vi "Create Frame Pattern Script.vi"(8 "error in (no error)":errorcluster, 10 "SPI_FRM_Config":T1 {"Addr" format="%x"; "Data" format="%x"}, 11 "SPI_Frame_Write in":refnum<class "SPI_Frame_Write.lvclass">) -> (0 "error out":errorcluster, 3 "SPI_Frame_Write out":refnum<class "SPI_Frame_Write.lvclass">)   [LabVIEW 2018, in "SPI_Frame_Write.lvclass"]
uses:
  SPI_Frame_Write.lvclass
  C:/P4 Workspace/PC Client/Solutions/5g_eap/HiSi/trunk/1.0/BML_Pattern_Gen_Refactor/SPI/SPI Frame Root/SPI_Frame_Root.lvclass
  Config Read SPI/SPI_FRM_Config.ctl
  Classes/Config_Read/RW_Option.ctl
  Config Read SPI/SPI_Mode.ctl
  SPI Frame Root/DataType.ctl
  Classes/BML_Frame_Root/Special Frame.ctl
  SPI Frame Root/SPI_Frame_Root.lvclass/SPI_Frame_Root.ctl
  Classes/BML_Frame_Root/BML_Frame_Root.lvclass
  SPI Frame Root/SPI_Frame_Root.lvclass
  Classes/Config_Read/Config_Read_BML.lvclass
  Config Read SPI/Config_Read_SPI.lvclass
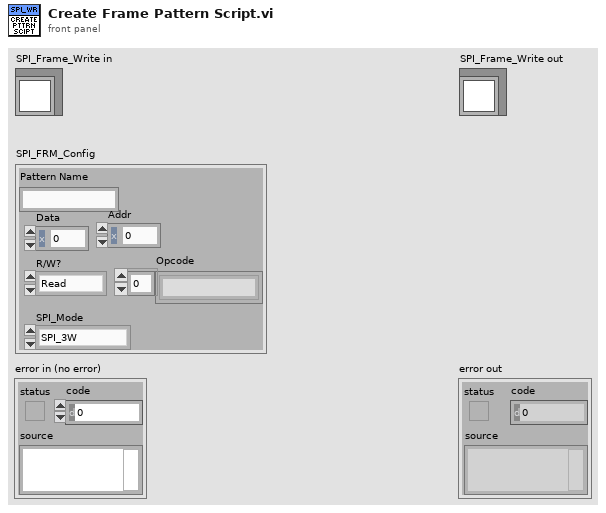
[diagram p1: front panel]
types:
  T1 = typedef "Config_Read_SPI.lvclass/SPI_FRM_Config.ctl" = cluster{"Pattern Name":string, "Data":u16, "Addr":u16, "R/W?":T2, "Opcode":string[], "SPI_Mode":T3}
  T2 = typedef "Config_Read_BML.lvclass/RW_Option.ctl" = enum16{"Read", "Write", "R/W"}
  T3 = typedef "Config_Read_SPI.lvclass/SPI_Mode.ctl" = enum16{"SPI_3W", "SPI_4W"}
  T4 = typedef "BML_Frame_Root.lvclass/Special Frame.ctl" = enum16{"Sync Header", "Protocol Header", "SW Trig", "SetID State", "Out SetID State", "SW Reset", "Wait", "SPI 4W FRM Start", "SPI 4W Wait", "SPI 4W FRM End", "SPI 4W Write Cmd", "SPI RD Collect Cmd", "SPI RD Value Cmd", "SPI 3W FRM Start", "SPI 3W Write Cmd", "SPI 3W FRM End", "SPI 3W Wait", "SPI 3W RD Cmd"}
  T5 = typedef "SPI_Frame_Root.lvclass/DataType.ctl" = enum16{"Drive", "Compare", "Read"}
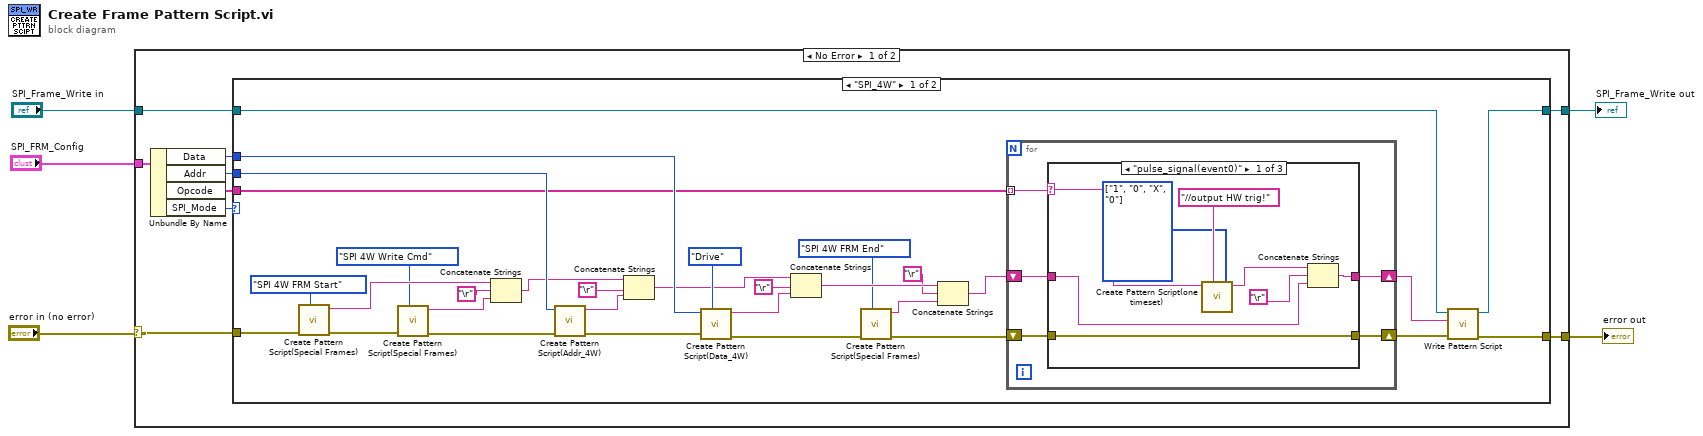
[diagram p0: block diagram]
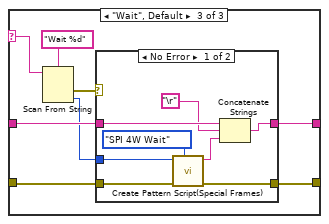
[diagram p3: hidden frame]
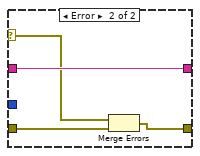
[diagram p4: hidden frame]
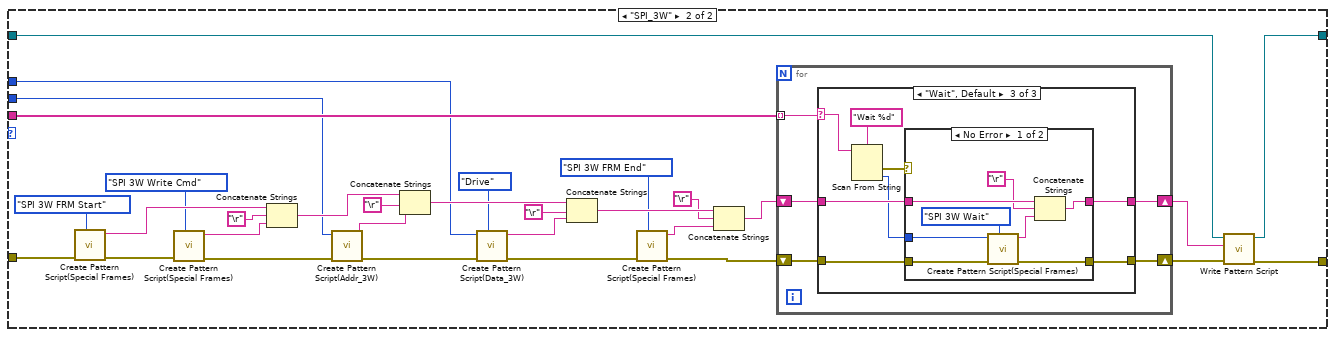
[diagram p5: hidden frame]
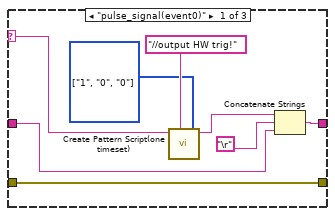
[diagram p6: hidden frame]
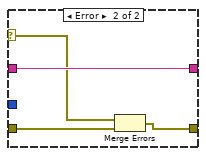
[diagram p8: hidden frame]
diagram:
  n1 = case shown="No Error" "error in (no error)" {
    selector: "error in (no error)" -> [w14 w147]
    tunnel: "SPI_Frame_Write in" -> [w9 w148]
    tunnel: [w8 w148] -> w3
    tunnel: [w10 w147] -> w2
    tunnel: "SPI_FRM_Config" -> [w13 _]
    frame No Error {
      n2 = Unbundle By Name(w13) -> ("Data"=w11:u16, "Addr"=w12:u16, "Opcode"=w7:string[], "SPI_Mode"=w6:T3)
      n3 = case shown="\"SPI_4W\"" w6 {
        tunnel: w14 -> [w45 w111]
        tunnel: w12 -> [w40 w89]
        tunnel: w11 -> [w34 w86]
        tunnel: [w29 w102] -> w10
        tunnel: w9 -> [w28 w101]
        tunnel: [w27 w100] -> w8
        tunnel: w7 -> [w20 w94]
        frame "SPI_4W" {
          n4 = call "Create Pattern Script(Special Frames).vi"("Special Frame Type"=Special_Frame."SPI 4W FRM Start", "error in (no error)"=w45) -> ("error out"=w44:errorcluster, "string out"=w43:string)  [unwired: 8 in]
          n5 = call "Create Pattern Script(Special Frames).vi"("Special Frame Type"=Special_Frame."SPI 4W Write Cmd", "error in (no error)"=w44) -> ("error out"=w39:errorcluster, "string out"=w41:string)  [unwired: 8 in]
          n6 = Concatenate Strings(w43, "\r", w41) -> (w38:string)
          n7 = call "Create Pattern Script(Addr_4W).vi"("error in (no error)"=w39, "Addr"=w40) -> ("error out"=w35:errorcluster, "String"=w36:string)  [unwired: 8 in]
          n8 = Concatenate Strings(w38, "\r", w36) -> (w32:string)
          n9 = call "Create Pattern Script(Data_4W).vi"("DataType"=DataType."Drive", "error in (no error)"=w35, "Data"=w34) -> ("error out"=w26:errorcluster, "String"=w30:string)  [unwired: 7 in]
          n10 = Concatenate Strings(w32, "\r", w30) -> (w24:string)
          n11 = call "Create Pattern Script(Special Frames).vi"("Special Frame Type"=Special_Frame."SPI 4W FRM End", "error in (no error)"=w26) -> ("error out"=w22:errorcluster, "string out"=w25:string)  [unwired: 8 in]
          n12 = Concatenate Strings(w24, "\r", w25) -> (w19:string)
          n13 = for {
            shift-right: [w47] -> w18
            shift-left: w19 -> [w50]
            shift-right: [w48] -> w21
            shift-left: w22 -> [w49]
            tunnel: w20 -> [w46] mode=indexing
            n14 = case shown="\"pulse_signal(event0)\"" w46 {
              selector: w46 -> [w55 _ w65]
              tunnel: w50 -> [w53 w60 w67]
              tunnel: w49 -> [w58 w59 w63]
              tunnel: [w52 w60 w68] -> w47
              tunnel: [w58 w59 w66] -> w48
              frame "pulse_signal(event0)" {
                w56 = enum16{"0", "1", "L", "H", "X", "V", "D", "M"}[] [enum."1", enum."0", enum."X", enum."0"] items=["0", "1", "L", "H", "X", "V", "D", "M"] ("PinState")
                n15 = call "Create Pattern Script(one timeset).vi"("Notes"="//output HW trig!", "PinState"=w56, "opcode"=w55) -> ("string out"=w51:string)  [unwired: 8 in]
                n16 = Concatenate Strings(w51, "\r", w53) -> (w52:string)
              }
              frame "" {
              }
              frame "Wait", Default {
                n17 = Scan From String(format string="Wait %d", input string=w65) -> (error out=w62:errorcluster, output 1=w61:i32)  [unwired: 3 in, 2 out]
                n18 = case shown="No Error" w62 {
                  selector: w62 -> [_ w79]
                  tunnel: [w76 w80] -> w68
                  tunnel: w67 -> [w75 w80]
                  tunnel: [w74 w77] -> w66
                  tunnel: w61 -> [w71 _]
                  tunnel: w63 -> [w70 w78]
                  frame No Error {
                    n19 = call "Create Pattern Script(Special Frames).vi"("Special Frame Type"=Special_Frame."SPI 4W Wait", "error in (no error)"=w70, "Num of Timeset"=w71) -> ("error out"=w74:errorcluster, "string out"=w73:string)  [unwired: 7 in]
                    n20 = Concatenate Strings(w75, "\r", w73) -> (w76:string)
                  }
                  frame Error {
                    n21 = Merge Errors(w79, w78) -> (w77:errorcluster)
                  }
                }
              }
            }
          }
          n22 = call "Write Pattern Script.vi"("error in (no error)"=w21, "Pattern Script"=w18, "SPI_Frame_Root in"=w28) -> ("error out"=w29:errorcluster, "SPI_Frame_Root out"=w27:refnum<class "SPI_Frame_Write.lvclass">)  [unwired: 7 in]
        }
        frame "SPI_3W" {
          n23 = call "Create Pattern Script(Special Frames).vi"("Special Frame Type"=Special_Frame."SPI 3W FRM Start", "error in (no error)"=w111) -> ("error out"=w110:errorcluster, "string out"=w109:string)  [unwired: 8 in]
          n24 = call "Create Pattern Script(Special Frames).vi"("Special Frame Type"=Special_Frame."SPI 3W Write Cmd", "error in (no error)"=w110) -> ("error out"=w88:errorcluster, "string out"=w107:string)  [unwired: 8 in]
          n25 = Concatenate Strings(w109, "\r", w107) -> (w106:string)
          n26 = call "Create Pattern Script(Addr_3W).vi"("error in (no error)"=w88, "Addr"=w89) -> ("error out"=w85:errorcluster, "String"=w87:string)  [unwired: 8 in]
          n27 = Concatenate Strings(w106, "\r", w87) -> (w104:string)
          n28 = call "Create Pattern Script(Data_3W).vi"("DataType"=DataType."Drive", "error in (no error)"=w85, "Data"=w86) -> ("error out"=w84:errorcluster, "String"=w83:string)  [unwired: 7 in]
          n29 = Concatenate Strings(w104, "\r", w83) -> (w98:string)
          n30 = call "Create Pattern Script(Special Frames).vi"("Special Frame Type"=Special_Frame."SPI 3W FRM End", "error in (no error)"=w84) -> ("error out"=w96:errorcluster, "string out"=w99:string)  [unwired: 8 in]
          n31 = Concatenate Strings(w98, "\r", w99) -> (w93:string)
          n32 = for {
            shift-right: [w113] -> w92
            shift-left: w93 -> [w116]
            shift-right: [w114] -> w95
            shift-left: w96 -> [w115]
            tunnel: w94 -> [w112] mode=indexing
            n33 = case shown="\"Wait\", Default" w112 {
              selector: w112 -> [w121 _ w131]
              tunnel: w116 -> [w119 w126 w133]
              tunnel: w115 -> [w124 w125 w129]
              tunnel: [w118 w126 w134] -> w113
              tunnel: [w124 w125 w132] -> w114
              frame "pulse_signal(event0)" {
                w122 = enum16{"0", "1", "L", "H", "X", "V", "D", "M"}[] [enum."1", enum."0", enum."0"] items=["0", "1", "L", "H", "X", "V", "D", "M"] ("PinState")
                n34 = call "Create Pattern Script(one timeset).vi"("Notes"="//output HW trig!", "PinState"=w122, "opcode"=w121) -> ("string out"=w117:string)  [unwired: 8 in]
                n35 = Concatenate Strings(w117, "\r", w119) -> (w118:string)
              }
              frame "" {
              }
              frame "Wait", Default {
                n36 = Scan From String(format string="Wait %d", input string=w131) -> (error out=w128:errorcluster, output 1=w127:i32)  [unwired: 3 in, 2 out]
                n37 = case shown="No Error" w128 {
                  selector: w128 -> [_ w145]
                  tunnel: [w142 w146] -> w134
                  tunnel: w133 -> [w141 w146]
                  tunnel: [w140 w143] -> w132
                  tunnel: w127 -> [w137 _]
                  tunnel: w129 -> [w136 w144]
                  frame No Error {
                    n38 = call "Create Pattern Script(Special Frames).vi"("Special Frame Type"=Special_Frame."SPI 3W Wait", "error in (no error)"=w136, "Num of Timeset"=w137) -> ("error out"=w140:errorcluster, "string out"=w139:string)  [unwired: 7 in]
                    n39 = Concatenate Strings(w141, "\r", w139) -> (w142:string)
                  }
                  frame Error {
                    n40 = Merge Errors(w145, w144) -> (w143:errorcluster)
                  }
                }
              }
            }
          }
          n41 = call "Write Pattern Script.vi"("error in (no error)"=w95, "Pattern Script"=w92, "SPI_Frame_Root in"=w101) -> ("error out"=w102:errorcluster, "SPI_Frame_Root out"=w100:refnum<class "SPI_Frame_Write.lvclass">)  [unwired: 7 in]
        }
      }
    }
    frame Error {
    }
  }
  "error out" <- w2
  "SPI_Frame_Write out" <- w3
